vi "PrepareProviderCall.vi"(6 "timeout in ms (-1)":i32, 8 "error in (no error)":errorcluster, 11 "ProviderCotentVI Path":path) -> (0 "error out":errorcluster)   [LabVIEW 2019, in "LabVIEW-VIProviderShell.lvlib" / "VIProviderShellHelper.lvclass"]
uses:
  VIProviderShellHelper.lvclass
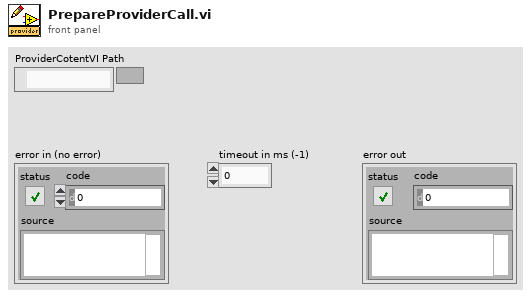
[diagram p1: front panel]
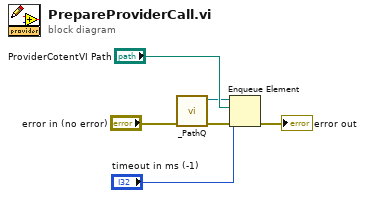
[diagram p0: block diagram]
diagram:
  n1 = call "_PathQ.vi"("error in (no error)"="error in (no error)") -> ("error out"=w2:errorcluster, "Queue out"=w4:refnum<queue>)  [unwired: 9 in]
  n2 = Enqueue Element(queue=w4, element="ProviderCotentVI Path", timeout in ms (-1)="timeout in ms (-1)", error in (no error)=w2) -> (error out=→"error out":errorcluster)  [unwired: 2 out]
